vi "Read Key.vi"(7 "data type":T1, 8 "error in (no error)":errorcluster, 9 "key":string, 10 "section":string, 11 "Configuration.lvclass in":refnum<class "Configuration.lvclass">) -> (0 "error out":errorcluster, 1 "found?":bool, 2 "Key":variant, 3 "Configuration.lvclass out":refnum<class "Configuration.lvclass">)   [LabVIEW 2011, in "Configuration.lvclass"]
uses:
  Configuration.lvclass
  Key Data Type.ctl
  Configuration.lvclass/Configuration.ctl
  <vilib>/Utility/config.llb/Read Key (Boolean).vi
  <vilib>/Utility/config.llb/Read Key (U32).vi
  <vilib>/Utility/config.llb/Read Key (I32).vi
  <vilib>/Utility/config.llb/Read Key (Double).vi
  <vilib>/Utility/config.llb/Read Key (String).vi
  <vilib>/Utility/config.llb/Read Key (Path).vi
  <vilib>/Utility/config.llb/NI_LVConfig.lvlib
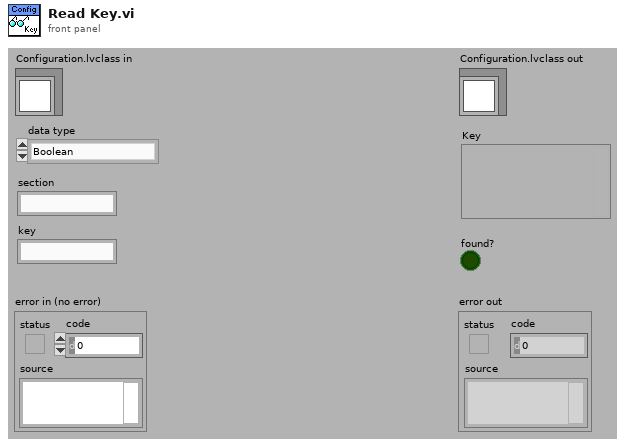
[diagram p1: front panel]
types:
  T1 = typedef "Configuration.lvclass/Key Data Type.ctl" = enum16{"Boolean", "U32", "I32", "Double", "String", "DAQmx Channel", "Path"}
  T2 = typedef "NI_LVConfig.lvlib/Config Data RefNum.ctl" = refnum<k1>
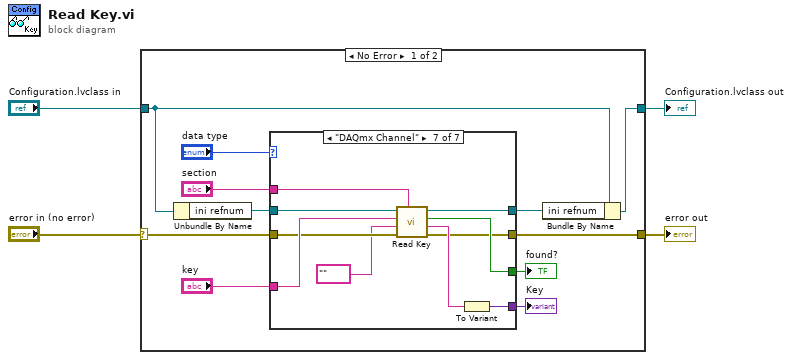
[diagram p0: block diagram]
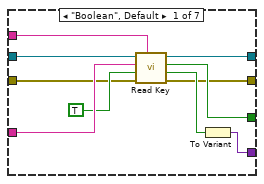
[diagram p2: hidden frame]
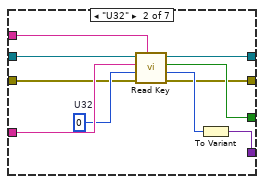
[diagram p3: hidden frame]
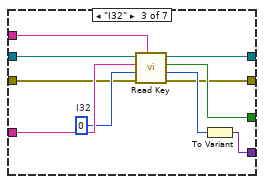
[diagram p4: hidden frame]
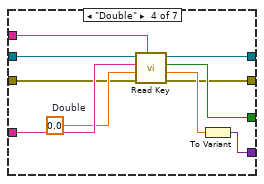
[diagram p5: hidden frame]
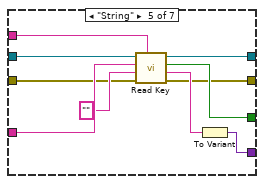
[diagram p6: hidden frame]
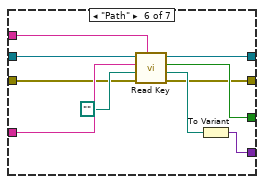
[diagram p7: hidden frame]
diagram:
  n1 = case shown="No Error" "error in (no error)" {
    selector: "error in (no error)" -> [w12 w86]
    tunnel: [w11 w86] -> w3
    tunnel: [w6 w87] -> w1
    tunnel: "Configuration.lvclass in" -> [w8 w87]
    frame No Error {
      n2 = Unbundle By Name(w8) -> ("ini refnum"=w15:T2)
      n3 = case shown="\"DAQmx Channel\"" "data type" {
        tunnel: "section" -> [w25 w35 w45 w55 w65 w75 w85]
        tunnel: w15 -> [w24 w34 w44 w54 w64 w74 w84]
        tunnel: [w23 w33 w43 w53 w63 w73 w83] -> w7
        tunnel: "key" -> [w22 w32 w42 w52 w62 w72 w82]
        tunnel: [w19 w31 w38 w48 w60 w70 w80] -> w10
        tunnel: [w21 w30 w40 w50 w59 w69 w79] -> w9
        tunnel: w12 -> [w17 w27 w37 w47 w57 w67 w78]
        tunnel: [w16 w26 w36 w46 w56 w66 w77] -> w11
        frame "Boolean", Default {
          n4 = call-poly <vilib>:"Read Key.vi"("section"=w25, "error in (no error)"=w17, "default value"=TRUE, "key"=w22, "refnum"=w24) -> ("error out"=w16:errorcluster, "value"=w20:bool, "found?"=w19:bool, "refnum out"=w23:T2)  [unwired: 3 in]
          n5 = To Variant(anything=w20) -> (Variant=w21:variant)
        }
        frame "U32" {
          w28 = u32 0  # U32
          n6 = call-poly <vilib>:"Read Key.vi"("section"=w35, "error in (no error)"=w27, "default value"=w28, "key"=w32, "refnum"=w34) -> ("error out"=w26:errorcluster, "value"=w29:u32, "found?"=w31:bool, "refnum out"=w33:T2)  [unwired: 3 in]
          n7 = To Variant(anything=w29) -> (Variant=w30:variant)
        }
        frame "I32" {
          w41 = 0  # I32
          n8 = call-poly <vilib>:"Read Key.vi"("section"=w45, "error in (no error)"=w37, "default value"=w41, "key"=w42, "refnum"=w44) -> ("error out"=w36:errorcluster, "value"=w39:i32, "found?"=w38:bool, "refnum out"=w43:T2)  [unwired: 3 in]
          n9 = To Variant(anything=w39) -> (Variant=w40:variant)
        }
        frame "Double" {
          w51 = 0.0  # Double
          n10 = call-poly <vilib>:"Read Key.vi"("section"=w55, "error in (no error)"=w47, "default value"=w51, "key"=w52, "refnum"=w54) -> ("error out"=w46:errorcluster, "value"=w49:dbl, "found?"=w48:bool, "refnum out"=w53:T2)  [unwired: 3 in]
          n11 = To Variant(anything=w49) -> (Variant=w50:variant)
        }
        frame "String" {
          n12 = call-poly <vilib>:"Read Key.vi"("section"=w65, "error in (no error)"=w57, "default value"="", "key"=w62, "refnum"=w64) -> ("error out"=w56:errorcluster, "value"=w58:string, "found?"=w60:bool, "refnum out"=w63:T2)  [unwired: 3 in]
          n13 = To Variant(anything=w58) -> (Variant=w59:variant)
        }
        frame "Path" {
          n14 = call-poly <vilib>:"Read Key.vi"("section"=w75, "error in (no error)"=w67, "default value"=path "", "key"=w72, "refnum"=w74) -> ("error out"=w66:errorcluster, "value"=w71:path, "found?"=w70:bool, "refnum out"=w73:T2)  [unwired: 3 in]
          n15 = To Variant(anything=w71) -> (Variant=w69:variant)
        }
        frame "DAQmx Channel" {
          n16 = call-poly <vilib>:"Read Key.vi"("section"=w85, "error in (no error)"=w78, "default value"=tag "" ("PID DAQmx Channels.S2"), "key"=w82, "refnum"=w84) -> ("error out"=w77:errorcluster, "value"=w81:string, "found?"=w80:bool, "refnum out"=w83:T2)  [unwired: 3 in]
          n17 = To Variant(anything=w81) -> (Variant=w79:variant)
        }
      }
      "found?" <- w10
      "Key" <- w9
      n18 = Bundle By Name(cluster=w8, "ini refnum"=w7) -> (w6:refnum<class "Configuration.lvclass">)
    }
    frame Error {
    }
  }
  "error out" <- w3
  "Configuration.lvclass out" <- w1
